vi "虚拟辐射监测仪-35-全屏版.vi"() -> ()   [LabVIEW 2013]
uses:
  <vilib>/registry/registry.llb/Registry RtKey.ctl
  <vilib>/Utility/xml.llb/Read From XML File(string).vi
  <vilib>/Instr/_visa.llb/VISA Configure Serial Port (Instr).vi
  <vilib>/Utility/inputDevices.llb/closeMouse.vi
  <vilib>/Utility/xml.llb/Write to XML File(string).vi
  <vilib>/Utility/inputDevices.llb/mouseAcquire.vi
  <vilib>/registry/registry.llb/Write Registry Value Simple STR.vi
  <vilib>/Utility/miscctls.llb/LVPoint32TypeDef.ctl
  <vilib>/Utility/miscctls.llb/LVPositionTypeDef.ctl
  <vilib>/Utility/miscctls.llb/LVBoundsTypeDef.ctl
panel:
  in  "实时数据":i32[](listbox)
  out "全探头窗口":refnum<vi>
  in  "更新列表？":bool
  out "测量值":dbl[](array[numeric])
  in  "切换窗口":bool
  in  "回复背景色标志":bool
  in  "等待时间（毫秒）":u32=10
  in  "T:G,F:B":bool
  in  "确认COM":bool
  in  "device ID":refnum<k1> caption="设备ID"
  in  "信号-弹窗选COM":bool
  out "菜单项":T1(ring)=enum."禁用"
  out "内容区域边界":T2
  out "内容区域位置":T3
  out "坐标":T4
  in  "开机启动":bool
  in  "收回":bool
  out "提示语":string
  in  "修改完成":bool=TRUE
  in  "变了？":bool
  out "编辑前项名":string[][](array[string])
  out "FREE":bool=TRUE
  in  "探头启用状态？":bool[](array[boolean])
  in  "报警记录标志？":bool[](array[boolean])
  in  "最大报警值":dbl[](array[numeric])
  in  "异常保存记录？":bool[](array[boolean])
  in  "发送次数":u8[](array[numeric])
  in  "暂停发送":bool=TRUE
  in  "探头地址":i32[](array[numeric])
  in  "备注信息":string[](array[string])
  in  "报警限值":dbl[](array[numeric])
  in  "报警状态？":bool[](array[boolean])
  out "退出":bool
  in  "波特率":enum16{"4800", "9600", "19200"}(ring)=enum."9600"
  out "报警记录":i32(listbox)
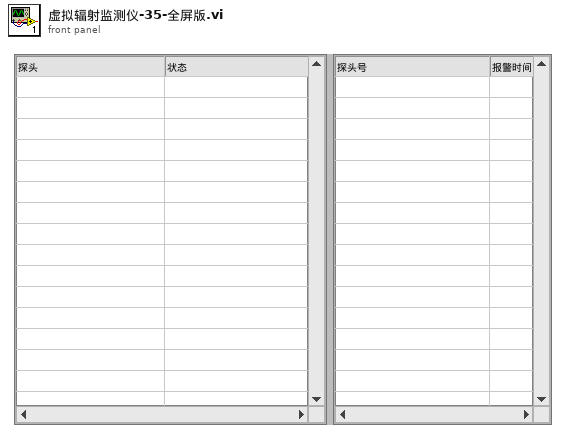
[diagram p1: front panel]
types:
  T1 = enum16{"启用", "禁用", "修改备注", "修改报警限值", "微调测量值", "探头排序", "备注信息", "报警限值"}
  T2 = typedef "LVBoundsTypeDef.ctl" = cluster{"Width":u32, "Height":u32}
  T3 = typedef "LVPositionTypeDef.ctl" = cluster{"Left":i32, "Top":i32}
  T4 = typedef "LVPoint32TypeDef.ctl" = cluster{"Horizontal":i32, "Vertical":i32}
  T5 = enum16{"初始化", "扫描探头", "发送命令", "接收数据", "暂停发送", "结束程序", "退出"}
  T6 = enum16{"启用", "禁用", "修改备注", "修改报警限值", "微调测量值", "探头排序", "备注信息"}
  T7 = enum32{"Invalid", "Standard", "Closed", "Hidden", "Minimized", "Maximized"}
  T8 = cluster{"测量值":refnum<vi>, "备注信息":refnum<vi>, "报警状态？":refnum<vi>, "探头启用状态？":refnum<vi>, "更新列表？":refnum<vi>}
  T9 = typedef "Registry RtKey.ctl" = enum32{"HKEY_CLASSES_ROOT", "HKEY_CURRENT_USER", "HKEY_LOCAL_MACHINE", "HKEY_USERS", "HKEY_PERFORMANCE_DATA", "HKEY_CURRENT_CONFIG", "HKEY_DYN_DATA"}
  T10 = cluster{"button 1":bool, "button 2":bool, "button 3":bool, "button 4":bool}
  T11 = typedef "LVRowAndColumnTypeDef.ctl" = cluster{"Row":i32, "Column":i32}
  T12 = cluster{"VISA":refnum<visa-resource-name>, "探头地址":i32[], "最大报警值":dbl[], "报警记录标志？":bool[], "报警状态？":bool[], "异常保存记录？":bool[], "报警限值":dbl[], "备注信息":string[], "探头启用状态？":bool[]}
  T13 = typedef "Registry refnum.ctl" = refnum<k1>
  T14 = cluster{"COM":refnum<visa-resource-name>, "探头地址":i32[], "探头启用状态？":bool[], "报警限值":dbl[], "开机启动？":bool, "备注信息":string[]}
  T15 = cluster{"COM":refnum<visa-resource-name>, "探头地址":i32[], "探头启用状态？":bool[], "开机启动？":bool, "探头信息":string[], "限值":cluster{"限值1":dbl, "限值2":dbl}[]}
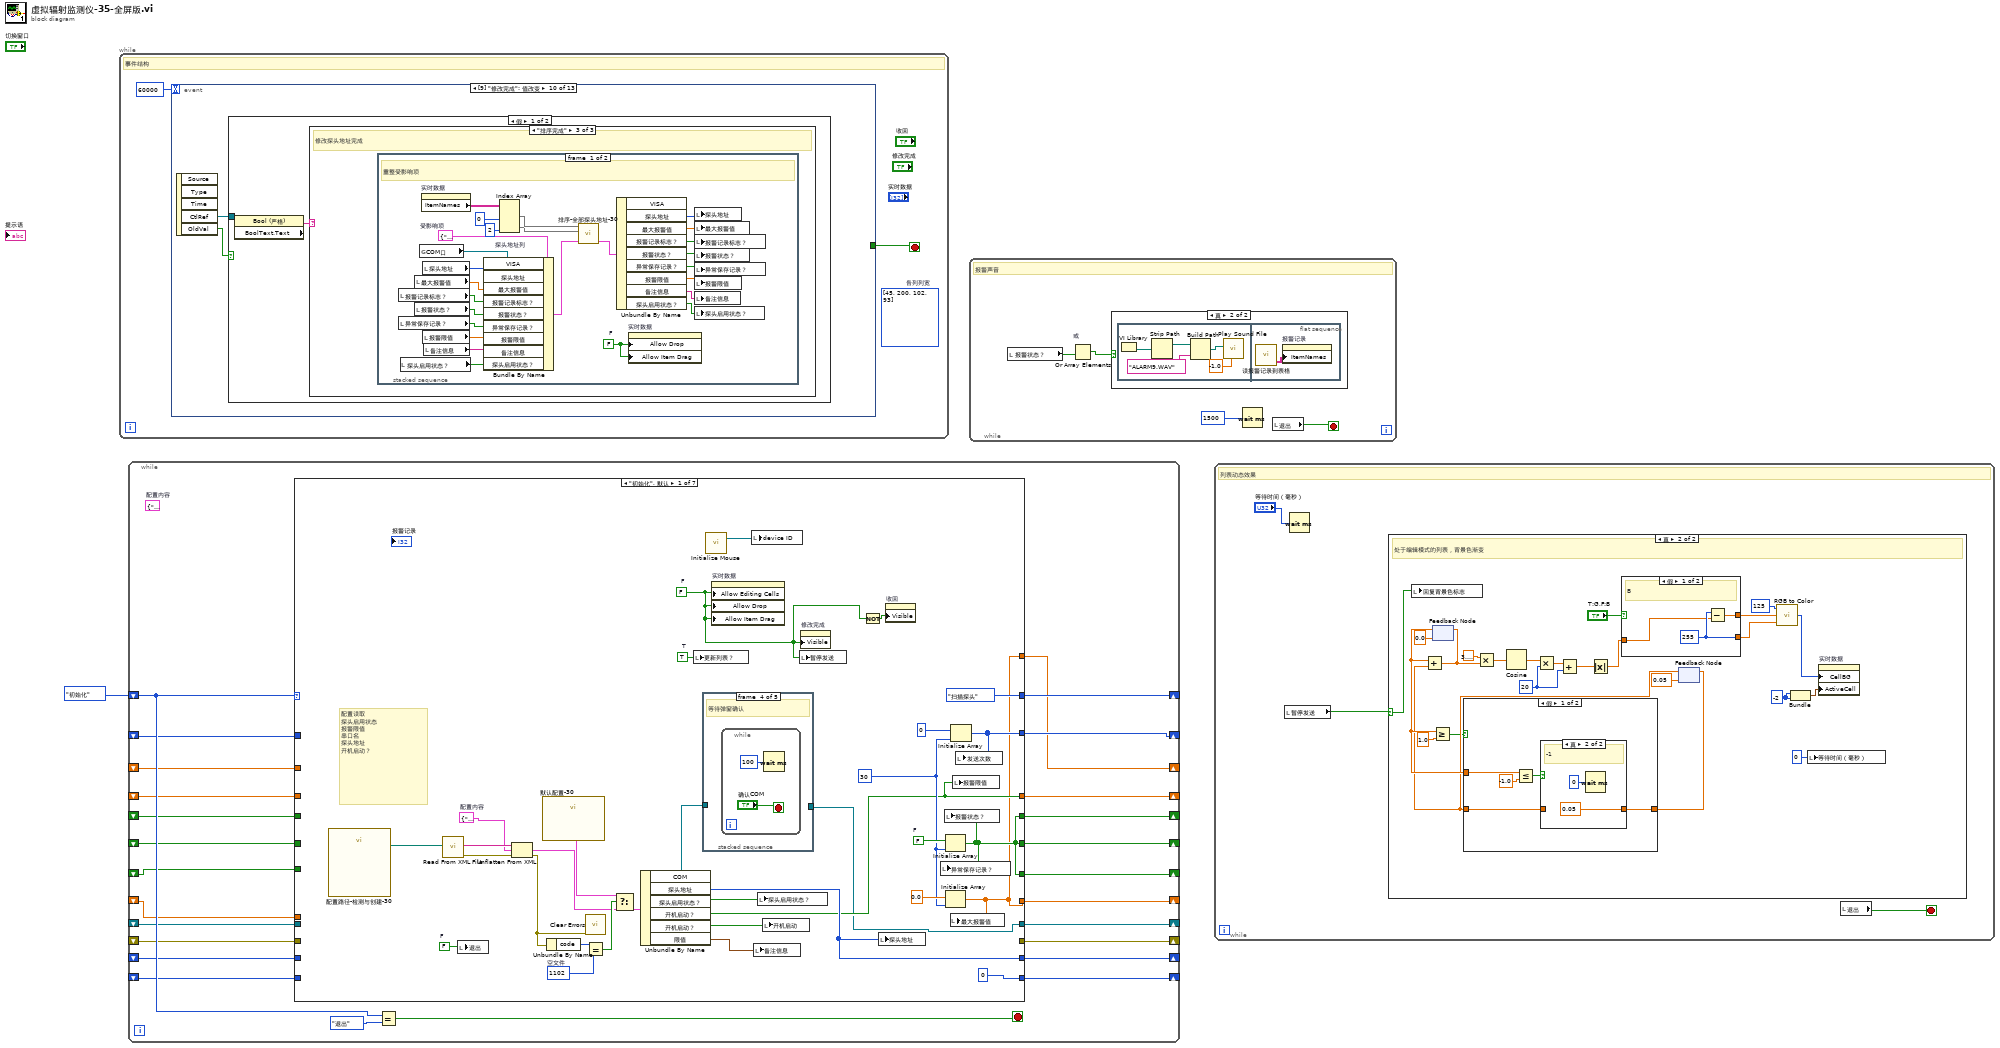
[diagram p0: block diagram]
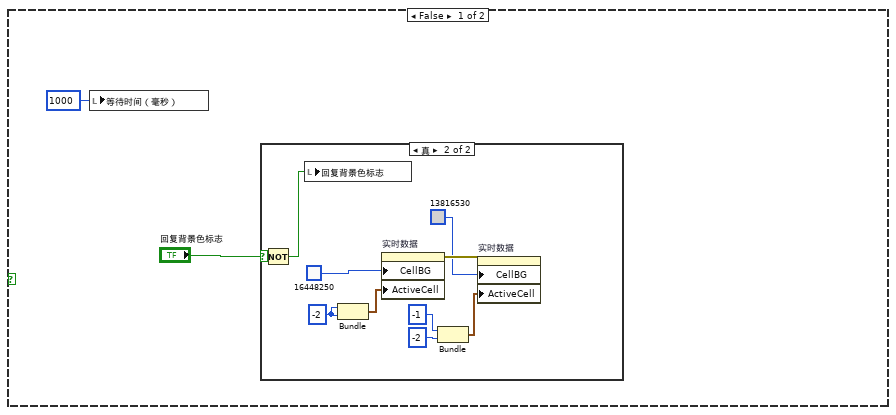
[diagram p2: hidden frame]
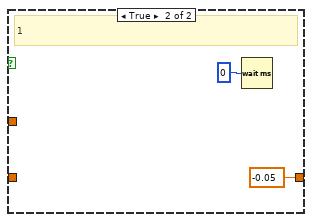
[diagram p5: hidden frame]
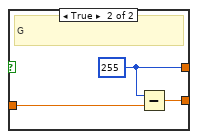
[diagram p6: hidden frame]
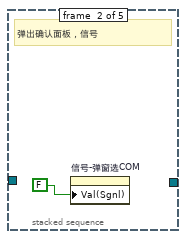
[diagram p8: hidden frame]
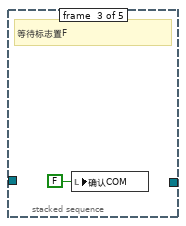
[diagram p9: hidden frame]
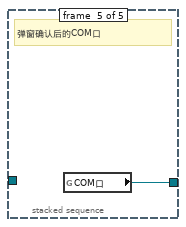
[diagram p10: hidden frame]
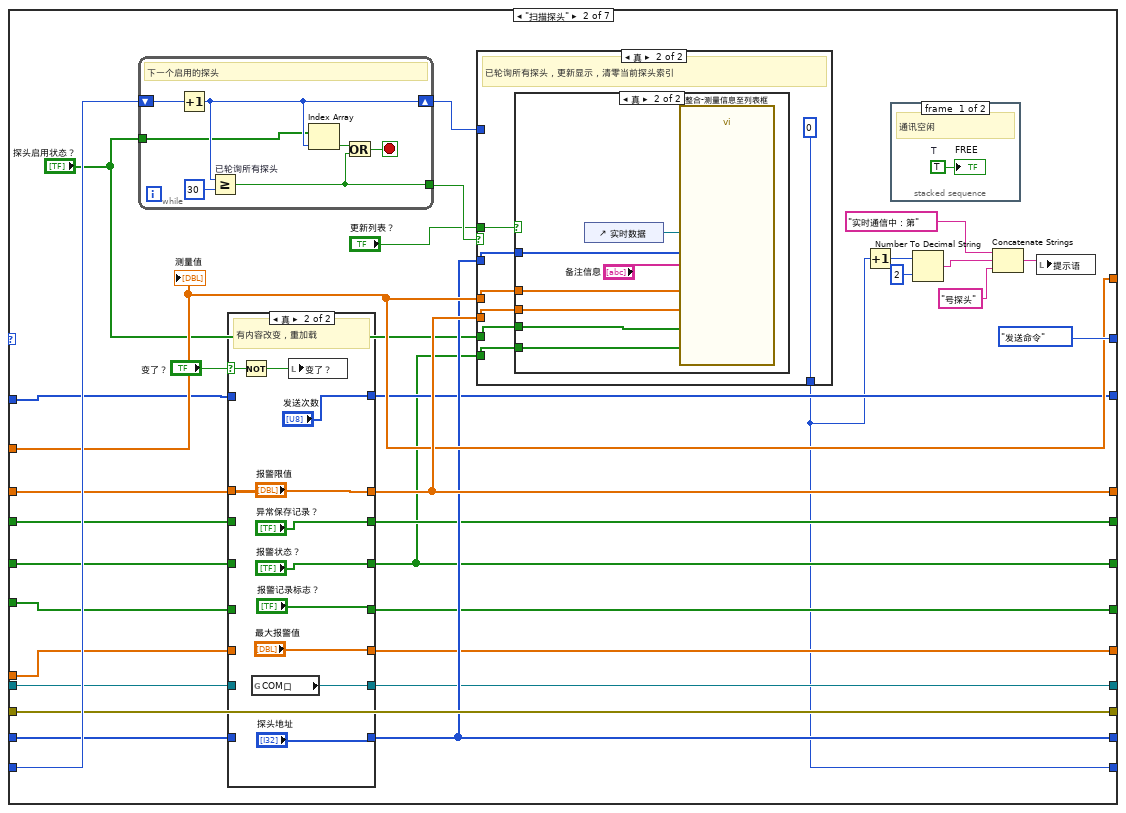
[diagram p11: hidden frame]
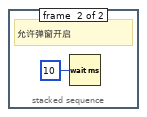
[diagram p13: hidden frame]
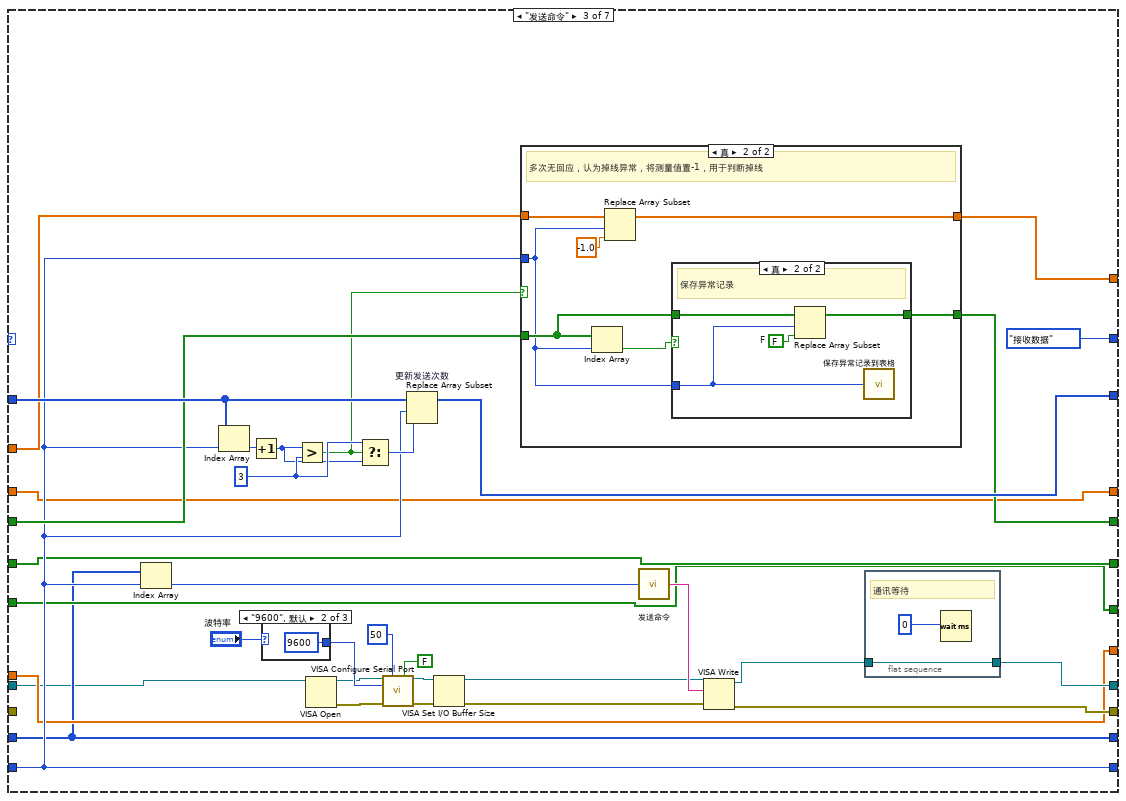
[diagram p16: hidden frame]
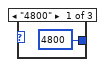
[diagram p19: hidden frame]
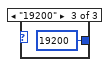
[diagram p20: hidden frame]
diagram:
  n1 = while {
    stop <- w3 stop-if-true
    (unwired) i32[] [45, 200, 102, 93]  # 各列列宽
    # "事件结构"
    n2 = event shown="[9] \"修改完成\": 值改变" {
      selector: _ -> [_ _ _ _ _ _ _ _ _ _ _ _ _]
      dyn-events: _ -> [_ _ _ _ _ _ _ _ _ _ _ _ _]
      timeout: 60000 -> [_ _ _ _ _ _ _ _ _ _ _ _ _]
      tunnel: [_ w4 _ _ _ _ _ _ _ _ _ _ _] -> w3
      event Timeout {
        n3 = event-data() -> ()  [unwired: 1 in, 2 out]
      }
      event Panel Close? {
        w4 = TRUE  # T
        n4 = event-data() -> ()  [unwired: 1 in, 4 out]
        n5 = event-data("Discard?"=w4) -> ()  [unwired: 1 in, 1 out]
        "退出" <- w4
      }
      event "信号-弹窗选COM": Value Change {
        n6 = event-data() -> ()  [unwired: 1 in, 6 out]
        n7 = flat-sequence {
          frame #0 {
            n8 = global read "全局变量-35点监测.vi" "COM口"() -> (w5:refnum<visa-resource-name>)
            n9 = control-ref of="本VI"() -> (w6:refnum<vi>)
            n10 = call "弹窗-提示选择Com口-30.vi"("VI引用句柄"=w6, "VISA资源名称"=w5) -> ()  [unwired: 9 in, 1 out]
          }
          frame #1 {
            n11 = local write "确认COM"(TRUE ("确认COM")) -> ()
          }
        }
      }
      event "实时数据": Mouse Move {
        # "注意：多列列表框一旦移动过\n就要重新定位坐标分界值"
        # "调试用"
        n12 = event-data() -> ("Coords"=w8:T4)  [unwired: 1 in, 4 out]
        n13 = disable-structure shown="禁用" {
          disable-tunnel: w8 -> [w11 _]
          frame Disabled {
            n14 = property on="实时数据" class="MCListbox (严格)"() -> ("ContentRectPos"=→"内容区域位置":T3, "ContentRectBounds"=→"内容区域边界":T2)  [unwired: 2 in, 2 out]
            "坐标" <- w11
          }
          frame Enabled {
          }
        }
      }
      event "实时数据": Mouse Down {
        # "使  右击行  列表能够获取焦点"
        n15 = event-data() -> ("Coords.Vertical"=w15:i32, "CtlRef"=w16:refnum<vi>)  [unwired: 1 in, 6 out]
        n16 = call-poly <vilib>:"Acquire Input Data.vi"("device ID"="device ID") -> ("button info"=w14:T10)  [unwired: 15 in, 3 out]
        n17 = Unbundle By Name(w14) -> ("button 2"=w13:bool)
        n18 = case shown="真" w13 {
          tunnel: w16 -> [_ w30]
          tunnel: w15 -> [_ w28]
          frame False {
          }
          frame True {
            w18 = TRUE  # T
            w26 = 20  # 行高
            # "右键"
            n19 = property class="多列列表框 (严格)"(reference=w30) -> ("ContentRectPosTop"=w29:i32)  [unwired: 1 in, 2 out]
            n20 = Subtract(x=w28, y=w29) -> (x-y=w27:i32)
            n21 = local read "实时数据"() -> (w19:i32[])
            n22 = Divide(x=w27, y=w26) -> (x/y=w25:dbl)
            n23 = Round Toward +Infinity(x=w25) -> (ceil(x): smallest int >= x=w24:dbl)
            n24 = To Long Integer(number=w24) -> (32bit integer=w22:i32)
            n25 = Subtract(x=w22, y=2 ("x")) -> (x-y=w20:i32)
            n26 = Build Array(w20) -> (w23:i32[])
            n27 = for {
              tunnel: w20 -> [w34]
              tunnel: w19 -> [w35] mode=indexing
              shift-right: [w31] -> w17
              shift-left: w18 -> [w32]
              stop <- w31 continue-if-true
              # "在选中项之外？"
              n28 = Not Equal?(x=w34, y=w35) -> (x != y?=w33:bool)
              n29 = And(x=w33, y=w32) -> (x .and. y?=w31:bool)
            }
            n30 = case shown="真" w17 {
              tunnel: w23 -> [_ w36]
              frame False {
                # "在已选中中，不赋值"
              }
              frame True {
                # "在选中项之外，赋值"
                n31 = local write "实时数据"(w36) -> ()
              }
            }
          }
        }
      }
      event "实时数据": Double Click {
        # "使 双击 可寻找到对应的列，并触发菜单处理事件，使打开修改弹窗"
        n32 = event-data() -> ("CtlRef"=w39:refnum<vi>, "Coords"=w40:T4)  [unwired: 1 in, 7 out]
        n33 = invoke class="多列列表框 (严格)" method="Point To Row Column"(reference=w39, "Point"=w40) -> ("CellPosition"=w38:T11)  [unwired: 5 in, 6 out]
        n34 = Unbundle By Name(w38) -> ("Column"=w37:i32)
        n35 = case shown="1" w37 {
          tunnel: [w42 T6."修改备注" ("菜单项") T6."微调测量值" ("菜单项") T6."修改报警限值" ("菜单项")] -> w41
          frame 0, Default {
            # "双击 探头地址列，禁用或启用"
            n36 = local read "探头启用状态？"() -> (w48:bool[])
            n37 = local read "实时数据"() -> (w47:i32[])
            n38 = Index Array(array=w47) -> (element=w46:i32)  [unwired: 1 in]
            n39 = Index Array(array=w48, index=w46) -> (element=w45:bool)
            n40 = Select(t=T6."禁用" ("菜单项"), s=w45, f=T6."启用" ("菜单项")) -> (s? t:f=w42:T6)
          }
          frame 1 {
            # "双击备注信息列，修改备注"
          }
          frame 2 {
            # "双击测量值列，微调探头"
          }
          frame 3 {
            # "双击报警限值列，修改限值"
          }
        }
        n41 = property on="菜单项" class="Enum (严格)"("Val(Sgnl)"=w41) -> ()  [unwired: 2 in, 2 out]
      }
      event "实时数据": Shortcut Menu Activation? {
        w58 = "修改备注" ("项名称")
        w61 = "禁用" ("项名称")
        w62 = "启用" ("项名称")
        n42 = event-data() -> ("CtlRef"=w70:refnum<vi>, "MenuRef"=w68:refnum<k9>)  [unwired: 1 in, 5 out]
        n43 = property class="多列列表框 (严格)"(reference=w70) -> ("Value"=w54:i32[])  [unwired: 1 in, 2 out]
        n44 = Array Size(array=w54) -> (size(s)=w56:i32)
        n45 = Equal?(x=w56, y=1) -> (x = y?=w63:bool)
        n46 = case shown="真" w63 {
          tunnel: [w72 w73] -> w65
          tunnel: [w72 w76] -> w64
          tunnel: w54 -> [_ w75]
          tunnel: [w71 w73] -> w57
          frame False {
            w72 = TRUE  # T
            # "多线选择"
            n47 = Not(x=w72) -> (.not. x?=w71:bool)
          }
          frame True {
            # "单项选择"
            n48 = local read "探头启用状态？"() -> (w77:bool[])
            n49 = Index Array(array=w75) -> (element=w74:i32)  [unwired: 1 in]
            n50 = Index Array(array=w77, index=w74) -> (element=w73:bool)
            n51 = Not(x=w73) -> (.not. x?=w76:bool)
          }
        }
        n52 = Set Menu Item Info(7:w62, 9:w64, 10:w62, 11:w68) -> (0:w67:errorcluster, 3:w66:refnum<k9>)  [unwired: 3 in]
        n53 = Set Menu Item Info(7:w61, 8:w67, 9:w65, 10:w61, 11:w66) -> (0:w60:errorcluster, 3:w59:refnum<k9>)  [unwired: 2 in]
        n54 = Set Menu Item Info(7:w58, 8:w60, 9:w57, 10:w58, 11:w59) -> ()  [unwired: 2 in, 2 out]
        n55 = local read "暂停发送"() -> (w52:bool)
        n56 = Empty Array?(array=w54) -> (empty?=w55:bool)
        n57 = Or(x=w55, y=w52) -> (x .or. y?=w53:bool)
        n58 = event-data("Discard?"=w53) -> ()  [unwired: 1 in, 1 out]
      }
      event "实时数据": Shortcut Menu Selection (User) {
        # "不在此事件中处理菜单事件"
        n59 = event-data() -> ("ItemTag"=w79:string)  [unwired: 1 in, 7 out]
        n60 = property on="菜单项" class="Enum (严格)"() -> ("Strings []"=w80:string[])  [unwired: 2 in, 2 out]
        n61 = for {
          tunnel: w80 -> [w84] mode=indexing
          tunnel: w79 -> [w83]
          tunnel: [w81] -> w78
          i -> [w81]
          stop <- w82 stop-if-true
          # "寻找匹配项"
          n62 = Equal?(x=w84, y=w83) -> (x = y?=w82:bool)
        }
        n63 = property on="菜单项" class="Enum (严格)"("Val(Sgnl)"=w78) -> ()  [unwired: 2 in, 2 out]
      }
      event "菜单项": Value Change {
        # "用于在鼠标操作 或 菜单操作 中 触发菜单事件"
        n64 = event-data() -> ("CtlRef"=w86:refnum<vi>)  [unwired: 1 in, 4 out]
        n65 = local read "暂停发送"() -> (w85:bool)
        n66 = case shown="假" w85 {
          tunnel: w86 -> [w89 _]
          frame False {
            # "暂停发送状态下，不允许产生菜单事件"
            n67 = property class="Enum (严格)"(reference=w89) -> ("RingText.Text"=w88:string)  [unwired: 1 in, 2 out]
            n68 = local read "探头地址"() -> (w91:i32[])
            n69 = local read "实时数据"() -> (w87:i32[])
            n70 = local read "备注信息"() -> (w90:string[])
            n71 = case shown="\"修改备注\"" w88 {
              tunnel: w87 -> [w94 w101 w108 w122 w136 _ _ _ _]
              tunnel: w91 -> [_ _ w107 w121 w135 _ _ _ _]
              tunnel: w90 -> [_ _ w106 _ _ _ _ _ _]
              frame "启用" {
                # "启用探头"
                n72 = local read "探头启用状态？"() -> (w93:bool[])
                n73 = for {
                  tunnel: w94 -> [w98] mode=indexing
                  shift-right: [w95] -> w92
                  shift-left: w93 -> [w96]
                  w97 = TRUE  # T
                  n74 = Replace Array Subset "更新 探头启用状态"(array=w96, new element=w97, index=w98) -> (w95:bool[])
                }
                n75 = local write "探头启用状态？"(w92) -> ()
              }
              frame "禁用" {
                # "禁用探头"
                n76 = local read "探头启用状态？"() -> (w100:bool[])
                n77 = for {
                  tunnel: w101 -> [w105] mode=indexing
                  shift-right: [w102] -> w99
                  shift-left: w100 -> [w103]
                  w104 = FALSE  # F
                  n78 = Replace Array Subset "更新 探头启用状态"(array=w103, new element=w104, index=w105) -> (w102:bool[])
                }
                n79 = local write "探头启用状态？"(w99) -> ()
              }
              frame "修改备注" {
                # "备注 只允许单项选择"
                n80 = for {
                  tunnel: w107 -> [w116]
                  tunnel: w106 -> [w110]
                  tunnel: w108 -> [w109] mode=indexing
                  n81 = Index Array(array=w116, index=w109) -> (element=w115:i32)
                  n82 = Index Array(array=w110, index=w109) -> (element=w114:string)
                  n83 = call "创建文本2"("探头地址"=w115, "当前备注信息"=w114) -> ("Result"=w113:string)  [unwired: 12 in, 1 out]
                  n84 = call "弹窗-提示修改备注-30.vi"("信息输入"=w113) -> ("新备注"=w111:string, "确定"=w112:bool)  [unwired: 16 in, 1 out]
                  n85 = case shown="真" w112 {
                    tunnel: w111 -> [_ w119]
                    tunnel: w110 -> [_ w120]
                    tunnel: w109 -> [_ w118]
                    frame False {
                      # "取消不修改"
                    }
                    frame True {
                      # "确定则修改"
                      n86 = Replace Array Subset(array=w120, new element=w119, index=w118) -> (w117:string[])
                      n87 = local write "备注信息"(w117) -> ()
                    }
                  }
                }
              }
              frame "修改报警限值" {
                # "允许批量修改"
                n88 = stacked-sequence {
                  tunnel: w122 -> [_ w130 _]
                  tunnel: w121 -> [_ w129 _]
                  frame #0 {
                    # "等到通讯空闲"
                    n89 = while {
                      stop <- w124 stop-if-true
                      # "等到通讯空闲"
                      n90 = local read "FREE"() -> (w124:bool)
                      n91 = Wait (ms)(milliseconds to wait=u32 1 ("等待时间（毫秒）")) -> ()  [unwired: 1 out]
                    }
                  }
                  frame #1 {
                    n92 = global read "全局变量-35点监测.vi" "COM口"() -> (w125:refnum<visa-resource-name>)
                    n93 = local read "报警限值"() -> (w128:dbl[])
                    n94 = control-ref of="本VI"() -> (w127:refnum<vi>)
                    n95 = call "修改-探头报警值-30.vi"("VI引用句柄"=w127, "VISA资源名称"=w125, "限值 i"=w128, "探头地址"=w129, "探头索引（列表值）"=w130) -> (1:w126)  [unwired: 5 in, 1 out]
                    n96 = local write "报警限值"(w126) -> ()
                  }
                  frame #2 {
                    # "FREE 置 F"
                    n97 = local write "FREE"(FALSE ("FREE")) -> ()
                    n98 = local write "变了？"(TRUE ("变？报警限值")) -> ()
                  }
                }
              }
              frame "微调测量值" {
                n99 = Index Array(array=w136) -> (element=w134:i32)  [unwired: 1 in]
                n100 = Index Array(array=w135, index=w134) -> (element=w133:i32)
                n101 = stacked-sequence {
                  tunnel: w133 -> [_ w140 _]
                  frame #0 {
                    # "等到 通讯空闲"
                    n102 = while {
                      stop <- w137 stop-if-true
                      # "等到通讯空闲"
                      n103 = local read "FREE"() -> (w137:bool)
                    }
                  }
                  frame #1 {
                    # "微调"
                    n104 = global read "全局变量-35点监测.vi" "COM口"() -> (w138:refnum<visa-resource-name>)
                    n105 = control-ref of="本VI"() -> (w139:refnum<vi>)
                    n106 = call "修改-微调探头测量值-30.vi"("VI引用句柄"=w139, "探头地址"=w140, "VISA资源名称"=w138) -> ()  [unwired: 8 in, 1 out]
                  }
                  frame #2 {
                    # "FREE 置 F"
                    n107 = local write "FREE"(FALSE ("FREE")) -> ()
                  }
                }
              }
              frame "探头排序" {
                # "进入可拖拽模式"
                n108 = stacked-sequence {
                  frame #0 {
                    w143 = TRUE  # T
                    # "暂停发送"
                    n109 = local write "暂停发送"(w143) -> ()
                    n110 = local write "T:G,F:B"(TRUE ("T:G,F:B")) -> ()
                  }
                  frame #1 {
                    w145 = TRUE  # T
                    # "开始拖拽"
                    n111 = property on="修改完成" class="Bool (严格)"("Visible"=w145) -> ()  [unwired: 2 in, 2 out]
                    n112 = property on="实时数据" class="多列列表框 (严格)"("Allow Drop"=w145, "Allow Item Drag"=w145) -> ()  [unwired: 2 in, 2 out]
                    n113 = property on="修改完成" class="Bool (严格)"("BoolText.Text"="排序完成" ("布尔文本.文本")) -> ()  [unwired: 2 in, 2 out]
                  }
                  frame #2 {
                    n114 = local write "提示语"("拖拽行进行探头排序" ("提示语")) -> ()
                  }
                }
              }
              frame "备注信息" {
                # "进入可编辑模式"
                n115 = stacked-sequence {
                  frame #0 {
                    w148 = TRUE  # T
                    # "暂停发送"
                    n116 = local write "暂停发送"(w148) -> ()
                    n117 = local write "T:G,F:B"(FALSE ("T:G,F:B")) -> ()
                  }
                  frame #1 {
                    w151 = TRUE  # T
                    # "开始编辑"
                    n118 = property on="实时数据" class="MCListbox (严格)"() -> ("ItemNames"=→"编辑前项名":string[][])  [unwired: 2 in, 2 out]
                    n119 = property on="实时数据" class="多列列表框 (严格)"("Allow Editing Cells"=w151) -> ()  [unwired: 2 in, 2 out]
                    n120 = property on="修改完成" class="Bool (严格)"("BoolText.Text"="编辑完成" ("布尔文本.文本")) -> ()  [unwired: 2 in, 2 out]
                    n121 = property on="修改完成" class="Bool (严格)"("Visible"=w151) -> ()  [unwired: 2 in, 2 out]
                  }
                  frame #2 {
                    n122 = local write "提示语"("点击备注信息单元格编辑" ("提示语")) -> ()
                  }
                }
              }
              frame "报警限值" {
                # "批量修改报警限值"
              }
              frame "假", Default {
              }
            }
          }
          frame True {
            # "暂停发送状态下，不允许产生菜单事件"
          }
        }
      }
      event "修改完成": Value Change {
        n123 = event-data() -> ("CtlRef"=w154:refnum<vi>, "OldVal"=w153:bool)  [unwired: 1 in, 3 out]
        n124 = case shown="假" w153 {
          tunnel: w154 -> [w156 _]
          frame False {
            n125 = property class="Bool (严格)"(reference=w156) -> ("BoolText.Text"=w155:string)  [unwired: 1 in, 2 out]
            n126 = case shown="\"排序完成\"" w155 {
              frame "假", Default {
              }
              frame "编辑完成" {
                # "修改备注信息完成"
                n127 = stacked-sequence {
                  frame #0 {
                    w158 = FALSE  # F
                    w162 = 1 ("禁用的索引 (列)")
                    # "更改受影响项"
                    n128 = property on="实时数据" class="MCListbox (严格)"() -> (error out=w161:errorcluster, "ItemNames"=w164:string[][])  [unwired: 2 in, 1 out]
                    n129 = local read "编辑前项名"() -> (w163:string[][])
                    n130 = Index Array "备注咧"(array=w164, index (col)=w162) -> (element=w159:string[])  [unwired: 1 in]
                    n131 = Replace Array Subset(array=w163, new element=w159, index (col)=w162) -> (w160:string[][])  [unwired: 1 in]
                    n132 = local write "备注信息"(w159) -> ()
                    n133 = property on="实时数据" class="MCListbox (严格)"(error in=w161, "ItemNames"=w160) -> (error out=w157:errorcluster)  [unwired: 1 in, 1 out]
                    n134 = property on="实时数据" class="MCListbox (严格)"(error in=w157, "Allow Editing Cells"=w158) -> ()  [unwired: 1 in, 2 out]
                  }
                  frame #1 {
                    # "更改标志，使在状态机中检测到更改"
                    n135 = flat-sequence {
                      frame #0 {
                        w165 = TRUE  # T
                        n136 = local write "变了？"(w165) -> ()
                      }
                      frame #1 {
                        w167 = FALSE  # F
                        w166 = FALSE  # F
                        n137 = local write "暂停发送"(w167) -> ()
                        n138 = property on="修改完成" class="Bool (严格)"("Visible"=w166) -> ()  [unwired: 2 in, 2 out]
                      }
                    }
                  }
                }
              }
              frame "排序完成" {
                # "修改探头地址完成"
                n139 = stacked-sequence {
                  frame #0 {
                    w173 = T12 {"VISA"="", "探头地址"=[], "最大报警值"=[], "报警记录标志？"=[], "报警状态？"=[], "异常保存记录？"=[], "报警限值"=[], "备注信息"=["4号楼509", "", "", "", "", "", "", "", "", "", "", "", "", "", "", "", "", "", "", "", "", "", "", "", "", "", "", "", "", ""], "探头启用状态？"=[]}  # 受影响项
                    w191 = FALSE  # F
                    # "重整受影响项"
                    n140 = local read "报警记录标志？"() -> (w187:bool[])
                    n141 = local read "异常保存记录？"() -> (w189:bool[])
                    n142 = local read "探头启用状态？"() -> (w172:bool[])
                    n143 = local read "最大报警值"() -> (w186:dbl[])
                    n144 = local read "报警状态？"() -> (w188:bool[])
                    n145 = global read "全局变量-35点监测.vi" "COM口"() -> (w169:refnum<visa-resource-name>)
                    n146 = property on="实时数据" class="MCListbox (严格)"() -> ("ItemNames"=w193:string[][])  [unwired: 2 in, 2 out]
                    n147 = local read "探头地址"() -> (w185:i32[])
                    n148 = local read "报警限值"() -> (w190:dbl[])
                    n149 = local read "备注信息"() -> (w176:string[])
                    n150 = Bundle By Name(cluster=w173, "VISA"=w169, "探头地址"=w185, "最大报警值"=w186, "报警记录标志？"=w187, "报警状态？"=w188, "异常保存记录？"=w189, "报警限值"=w190, "备注信息"=w176, "探头启用状态？"=w172) -> (w184:T12)
                    n151 = Index Array "探头地址列"(array=w193, index (col) #1=0 ("禁用的索引 (列)"), index (col) #2=2 ("索引 (列)")) -> (element #1=w175:string[], element #2=w174:string[])  [unwired: 2 in]
                    n152 = call "排序-全部探头地址-30.vi"("受影响项i"=w184, "备注信息列"=w174, "探头序号列"=w175) -> ("受影响项o"=w183:T12)  [unwired: 8 in]
                    n153 = Unbundle By Name(w183) -> ("探头地址"=w182:i32[], "最大报警值"=w181:dbl[], "报警记录标志？"=w180:bool[], "报警状态？"=w179:bool[], "异常保存记录？"=w178:bool[], "报警限值"=w177:dbl[], "备注信息"=w171:string[], "探头启用状态？"=w170:bool[])  [unwired: 1 out]
                    n154 = property on="实时数据" class="多列列表框 (严格)"("Allow Drop"=w191, "Allow Item Drag"=w191) -> ()  [unwired: 2 in, 2 out]
                    n155 = local write "备注信息"(w171) -> ()
                    n156 = local write "探头启用状态？"(w170) -> ()
                    n157 = local write "探头地址"(w182) -> ()
                    n158 = local write "最大报警值"(w181) -> ()
                    n159 = local write "报警记录标志？"(w180) -> ()
                    n160 = local write "报警状态？"(w179) -> ()
                    n161 = local write "异常保存记录？"(w178) -> ()
                    n162 = local write "报警限值"(w177) -> ()
                  }
                  frame #1 {
                    # "更改标志，使在状态机中检测到更改"
                    n163 = flat-sequence {
                      frame #0 {
                        w194 = TRUE  # T
                        n164 = local write "变了？"(w194) -> ()
                      }
                      frame #1 {
                        w196 = FALSE  # F
                        w195 = FALSE  # F
                        n165 = local write "暂停发送"(w196) -> ()
                        n166 = property on="修改完成" class="Bool (严格)"("Visible"=w195) -> ()  [unwired: 2 in, 2 out]
                      }
                    }
                  }
                }
              }
            }
          }
          frame True {
          }
        }
      }
      event "切换窗口": Value Change {
        n167 = event-data() -> ("OldVal"=w197:bool)  [unwired: 1 in, 5 out]
        n168 = case shown="真" w197 {
          frame False {
          }
          frame True {
            # "切换到大窗口浏览模式"
            n169 = control-ref of="探头启用状态？"() -> (w205:refnum<vi>)
            n170 = control-ref of="更新列表？"() -> (w198:refnum<vi>)
            n171 = control-ref of="本VI"() -> (w201:refnum<vi>)
            n172 = control-ref of="测量值"() -> (w219:refnum<vi>)
            n173 = control-ref of="备注信息"() -> (w218:refnum<vi>)
            n174 = control-ref of="报警状态？"() -> (w217:refnum<vi>)
            n175 = Bundle By Name(cluster=T8 {"测量值"=refnum, "备注信息"=refnum, "报警状态？"=refnum, "探头启用状态？"=refnum, "更新列表？"=refnum}, "测量值"=w219, "备注信息"=w218, "报警状态？"=w217, "更新列表？"=w198, "探头启用状态？"=w205) -> (w215:T8)
            n176 = vi-ref "探头模块-精简版.vi"() -> (w216:refnum<vi>)
            n177 = invoke on="传入引用" class="VI" method="Ctrl Val.Set"(reference=w216, "Control Name"="引用传入" ("控件名"), "Value"=w215) -> (reference out=w211:refnum<vi>, error out=w209:errorcluster)  [unwired: 2 in, 3 out]
            n178 = local write "更新列表？"(FALSE ("更新列表？")) -> ()
            n179 = invoke on="运行VI" class="VI" method="Run VI"(reference=w211, error in=w209, "Wait until done"=FALSE ("结束前等待"), "Auto Dispose Ref"=TRUE ("自动销毁引用")) -> (reference out=w210:refnum<vi>, error out=w206:errorcluster)  [unwired: 1 in, 3 out]
            n180 = invoke on="打开前面板" class="VI" method="FP.Open"(reference=w210, error in=w206, "Activate"=TRUE ("激活？"), "State"=T7."Standard" ("状态")) -> (reference out=→"全探头窗口":refnum<vi>, error out=w204:errorcluster)  [unwired: 1 in, 3 out]
            n181 = property class="VI"(reference=w201, error in=w204, "FP.State"=T7."Hidden" ("前面板窗口:状态")) -> (error out=w203:errorcluster)  [unwired: 1 out]
            n182 = call <vilib>:"Clear Errors.vi"("error in (no error)"=w203) -> ()  [unwired: 6 in, 1 out]
          }
        }
      }
      event "更新列表？": Value Change {
        n183 = event-data() -> ()  [unwired: 1 in, 6 out]
        n184 = local read "全探头窗口"() -> (w227:refnum<vi>)
        n185 = control-ref of="本VI"() -> (w224:refnum<vi>)
        n186 = disable-structure shown="启用" {
          disable-tunnel: w227 -> [w230 w231]
          disable-tunnel: [w229 w231] -> w226
          disable-tunnel: [w228 _] -> w225
          frame Disabled {
            n187 = invoke class="VI" method="Abort VI"(reference=w230) -> (reference out=w229:refnum<vi>, error out=w228:errorcluster)  [unwired: 2 in, 1 out]
          }
          frame Enabled {
          }
        }
        n188 = invoke class="VI" method="FP.Close"(reference=w226, error in=w225) -> (error out=w222:errorcluster)  [unwired: 1 in, 2 out]
        n189 = property class="VI"(reference=w224, error in=w222, "FP.State"=T7."Standard" ("前面板窗口:状态")) -> (error out=w221:errorcluster)  [unwired: 1 out]
        n190 = call <vilib>:"Clear Errors.vi"("error in (no error)"=w221) -> ()  [unwired: 6 in, 1 out]
      }
      event "开机启动": Value Change {
        n191 = event-data() -> ()  [unwired: 1 in, 5 out]
        n192 = case shown="真" "开机启动" {
          frame False {
            n193 = call <vilib>:"Open Registry Key.vi"("subkey"="SOFTWARE\\Microsoft\\Windows\\CurrentVersion\\Run", "root key (HKEY_LOCAL_MACHINE)"=Registry_RtKey."HKEY_LOCAL_MACHINE") -> ("error out"=w238:errorcluster, "refnum out"=w239:T13)  [unwired: 8 in]
            n194 = call <vilib>:"Delete Registry Value.vi"("error in (no error)"=w238, "value"="6103J-16", "refnum"=w239) -> ("error out"=w237:errorcluster, "refnum out"=w236:T13)  [unwired: 7 in]
            n195 = call <vilib>:"Close Registry Key.vi"("error in (no error)"=w237, "refnum"=w236) -> ("error out"=w233:errorcluster)  [unwired: 5 in]
            n196 = call <vilib>:"Simple Error Handler.vi"("error in (no error)"=w233) -> ()  [unwired: 4 in, 5 out]
          }
          frame True {
            n197 = VI Library() -> (path=w243:path)
            n198 = Strip Path(path=w243) -> (stripped path=w245:path)  [unwired: 1 out]
            n199 = call <vilib>:"Create Registry Key.vi"("subkey"="SOFTWARE\\Microsoft\\Windows\\CurrentVersion\\Run", "root key (HKEY_LOCAL_MACHINE)"=Registry_RtKey."HKEY_LOCAL_MACHINE") -> ("refnum out"=w252:T13)  [unwired: 7 in, 2 out]
            n200 = Build Path(base path=w245, name or relative path="核辐射在线测量16路.exe" ("读报警文件")) -> (appended path=w242:path)
            n201 = Path To String(path=w242) -> (string=w241:string)
            n202 = call-poly <vilib>:"Write Registry Value Simple.vi"("String/Binary data"=w241, "simple data type"=enum16{"String", "Binary", "DWORD"}."String", "value"="6103J-16", "refnum"=w252) -> ("error out"=w247:errorcluster, "refnum out"=w248:T13)  [unwired: 4 in]
            n203 = call <vilib>:"Close Registry Key.vi"("error in (no error)"=w247, "refnum"=w248) -> ("error out"=w249:errorcluster)  [unwired: 5 in]
            n204 = call <vilib>:"Simple Error Handler.vi"("error in (no error)"=w249) -> ()  [unwired: 4 in, 5 out]
          }
        }
      }
    }
  }
  n205 = while {
    shift-right: [w277] -> _
    shift-left: T5."初始化" -> [w278]
    shift-right: [w276] -> _
    shift-left: _ -> [w274]
    shift-right: [w275] -> _
    shift-left: _ -> [w273]
    shift-right: [w258] -> _
    shift-left: _ -> [w263]
    shift-right: [w257] -> _
    shift-left: _ -> [w265]
    shift-right: [w262] -> _
    shift-left: _ -> [w264]
    shift-right: [w270] -> _
    shift-left: _ -> [w271]
    shift-right: [w254] -> _
    shift-left: _ -> [w268]
    shift-right: [w266] -> _
    shift-left: _ -> [w267]
    shift-right: [w256] -> _
    shift-left: _ -> [w261]
    shift-right: [w255] -> _
    shift-left: _ -> [w260]
    shift-right: [w259] -> _
    shift-left: _ -> [w269]
    stop <- w279 stop-if-true
    (unwired) T14 {"COM"="", "探头地址"=[], "探头启用状态？"=[], "报警限值"=[], "开机启动？"=FALSE, "备注信息"=[]}  # 配置内容
    n206 = case shown="\"初始化\", 默认" w278 {
      selector: w278 -> [_ _ _ _ _ _ w584]
      tunnel: [T5."扫描探头" T5."发送命令" T5."接收数据" T5."暂停发送" w551 T5."退出" w584] -> w277
      tunnel: [w281 w326 w401 w461 w549 _ w583] -> w276
      tunnel: [_ w347 w413 w460 w548 _ w582] -> w275
      tunnel: w274 -> [_ w327 w391 w463 w549 w569 w583]
      tunnel: w273 -> [_ w347 _ w462 w548 w571 w582]
      tunnel: w271 -> [_ w332 w408 w457 w541 w562 w578]
      tunnel: [w288 w331 w406 w451 w541 w562 w578] -> w270
      tunnel: w269 -> [_ w340 w392 w445 w535 w556 w574]
      tunnel: w268 -> [_ w348 w400 w444 w534 w555 w573]
      tunnel: w267 -> [_ w334 w405 w456 w539 w560 w575]
      tunnel: [w287 w333 w404 w450 w539 w560 w575] -> w266
      tunnel: [0 ("维数大小") w319 w400 w444 w534 w555 w573] -> w254
      tunnel: w265 -> [_ w330 w395 w458 w538 w559 w581]
      tunnel: w264 -> [_ w341 w398 w455 w542 w563 w577]
      tunnel: w263 -> [_ w342 w396 w449 w540 w561 w576]
      tunnel: [w286 w341 w397 w452 w542 w563 w577] -> w262
      tunnel: w261 -> [_ w336 w394 w454 w537 w558 w580]
      tunnel: w260 -> [_ w338 w393 w453 w536 w557 w579]
      tunnel: [w292 w339 w392 w445 w535 w556 w574] -> w259
      tunnel: [w289 w343 w396 w449 w540 w561 w576] -> w258
      tunnel: [w287 w329 w395 w447 w538 w559 w581] -> w257
      tunnel: [w287 w335 w394 w448 w537 w558 w580] -> w256
      tunnel: [w286 w337 w393 w446 w536 w557 w579] -> w255
      frame "初始化", Default {
        w280 = TRUE  # T
        w284 = FALSE  # F
        w291 = T14 {"COM"="", "探头地址"=[], "探头启用状态？"=[], "报警限值"=[], "开机启动？"=FALSE, "备注信息"=[]}  # 配置内容
        w298 = 1102  # 空文件
        w300 = 30 ("维数大小")
        w304 = FALSE  # F
        w310 = FALSE  # F
        # "配置读取\n探头启用状态\n报警限值\n串口名\n探头地址\n开机启动？"
        n207 = call "配置路径-检测与创建-30.vi"() -> ("配置文件路径"=w309:path)  [unwired: 11 in]
        n208 = call-poly <vilib>:"Read From XML File.vi"("XML File Path"=w309) -> ("error out"=w307:errorcluster, "XML Elements"=w308:string)  [unwired: 8 in, 1 out]
        n209 = local write "退出"(w310) -> ()
        n210 = Unflatten From XML(xml string=w308, type=w291, error in (no error)=w307) -> (value=w294:T14, error out=w293:errorcluster)
        n211 = call "默认配置-30.vi"() -> ("默认配置"=w295:T15)  [unwired: 11 in]
        n212 = Unbundle By Name(w293) -> ("code"=w299:i32)
        n213 = call <vilib>:"Clear Errors.vi"("error in (no error)"=w293) -> ()  [unwired: 6 in, 1 out]
        n214 = Equal?(x=w299, y=w298) -> (x = y?=w296:bool)
        n215 = Select(t=w295, s=w296, f=w294) -> (s? t:f=w297:T15)
        n216 = Unbundle By Name(w297) -> ("COM"=w282:refnum<visa-resource-name>, "探头地址"=w292:i32[], "探头启用状态？"=w305:bool[], "开机启动？"=w289:bool, "开机启动？"=w306:bool, "限值"=w290:cluster{"限值1":dbl, "限值2":dbl}[])
        n217 = local write "更新列表？"(w280) -> ()
        n218 = stacked-sequence {
          tunnel: w282 -> [_ _ _ _ _]
          tunnel: [_ _ _ _ w316] -> w281
          frame #0 {
            # "读取配置保存的COM口"
          }
          frame #1 {
            # "弹出确认面板，信号"
            n219 = property on="信号-弹窗选COM" class="Bool (严格)"("Val(Sgnl)"=FALSE ("允许编辑单元格")) -> ()  [unwired: 2 in, 2 out]
          }
          frame #2 {
            # "等待标志置F"
            n220 = local write "确认COM"(FALSE ("确认COM")) -> ()
          }
          frame #3 {
            # "等待弹窗确认"
            n221 = while {
              stop <- "确认COM" stop-if-true
              n222 = Wait (ms)(milliseconds to wait=u32 100 ("等待时间（毫秒）")) -> ()  [unwired: 1 out]
            }
          }
          frame #4 {
            # "弹窗确认后的COM口"
            n223 = global read "全局变量-35点监测.vi" "COM口"() -> (w316:refnum<visa-resource-name>)
          }
        }
        n224 = call <vilib>:"Initialize Mouse.vi"() -> ("device ID"=w285:refnum<k1>)  [unwired: 10 in, 1 out]
        n225 = property on="实时数据" class="多列列表框 (严格)"("Allow Editing Cells"=w284, "Allow Drop"=w284, "Allow Item Drag"=w284) -> ()  [unwired: 2 in, 2 out]
        n226 = local write "device ID"(w285) -> ()
        n227 = local write "备注信息"(w290) -> ()
        n228 = local write "探头启用状态？"(w305) -> ()
        n229 = local write "开机启动"(w306) -> ()
        n230 = local write "暂停发送"(w284) -> ()
        n231 = property on="修改完成" class="Bool (严格)"("Visible"=w284) -> ()  [unwired: 2 in, 2 out]
        n232 = Not(x=w284) -> (.not. x?=w283:bool)
        n233 = local write "探头地址"(w292) -> ()
        n234 = property on="收回" class="Bool (严格)"("Visible"=w283) -> ()  [unwired: 2 in, 2 out]
        n235 = Initialize Array(w304, w300) -> (w287:bool[])
        n236 = local write "异常保存记录？"(w287) -> ()
        n237 = local write "报警状态？"(w287) -> ()
        n238 = Initialize Array(0.0 ("维数大小"), w300) -> (w286:dbl[])
        n239 = local write "最大报警值"(w286) -> ()
        n240 = Initialize Array(u8 0 ("维数大小"), w300) -> (w288:u8[])
        n241 = local write "报警限值"(w289) -> ()
        n242 = local write "发送次数"(w288) -> ()
      }
      frame "扫描探头" {
        n243 = while {
          shift-right: [w386] -> w346
          shift-left: w348 -> [w390]
          tunnel: [w385] -> w318
          tunnel: "探头启用状态？" -> [w384]
          stop <- w387 stop-if-true
          # "下一个启用的探头"
          n244 = Increment(x=w390) -> (x+1=w386:i32)
          n245 = Greater Or Equal? "已轮询所有探头"(x=w386, y=u8 30) -> (x >= y?=w385:bool)
          n246 = Index Array(array=w384, index=w386) -> (element=w389:bool)
          n247 = Or(x=w389, y=w385) -> (x .or. y?=w387:bool)
        }
        n248 = case shown="真" "变了？" {
          selector: "变了？" -> [_ w365]
          tunnel: [w356 "报警限值"] -> w343
          tunnel: w342 -> [w356 _]
          tunnel: w340 -> [w355 _]
          tunnel: [w355 "探头地址"] -> w339
          tunnel: w338 -> [w354 _]
          tunnel: [w354 "最大报警值"] -> w337
          tunnel: w336 -> [w353 _]
          tunnel: [w353 "报警记录标志？"] -> w335
          tunnel: w330 -> [w352 _]
          tunnel: [w352 "报警状态？"] -> w329
          tunnel: w334 -> [w351 _]
          tunnel: [w351 "异常保存记录？"] -> w333
          tunnel: w332 -> [w350 _]
          tunnel: [w350 "发送次数"] -> w331
          tunnel: w327 -> [w349 _]
          tunnel: [w349 w357] -> w326
          frame False {
            # "没有内容改变，则传递"
          }
          frame True {
            # "有内容改变，重加载"
            n249 = Not(x=w365) -> (.not. x?=w364:bool)
            n250 = global read "全局变量-35点监测.vi" "COM口"() -> (w357:refnum<visa-resource-name>)
            n251 = local write "变了？"(w364) -> ()
          }
        }
        n252 = case shown="真" w318 {
          tunnel: w341 -> [_ w376]
          tunnel: w343 -> [_ w375]
          tunnel: w329 -> [_ w374]
          tunnel: w339 -> [_ w373]
          tunnel: w346 -> [w369 _]
          tunnel: [w369 u8 0] -> w319
          tunnel: "探头启用状态？" -> [_ w371]
          tunnel: "更新列表？" -> [_ w370]
          frame False {
            # "更新当前探头索引，通知全探头窗口更新显示"
          }
          frame True {
            # "已轮询所有探头，更新显示，清零当前探头索引"
            n253 = case shown="真" w370 {
              tunnel: w376 -> [_ w381]
              tunnel: w375 -> [_ w380]
              tunnel: w374 -> [_ w379]
              tunnel: w373 -> [_ w378]
              tunnel: w371 -> [_ w377]
              frame False {
              }
              frame True {
                n254 = control-ref of="实时数据"() -> (w383:refnum<vi>)
                n255 = call "整合-测量信息至列表框.vi"("限值"=w379, "测量值"=w377, "MCListbox引用句柄"=w383, "备注信息"=w380, "报警状态"=w381, "探头地址"="备注信息", "探头启用状态？"=w378) -> ()  [unwired: 5 in]
              }
            }
          }
        }
        n256 = Increment(x=w319) -> (x+1=w320:i32)
        n257 = stacked-sequence {
          frame #0 {
            w367 = TRUE  # T
            # "通讯空闲"
            "FREE" <- w367
          }
          frame #1 {
            # "允许弹窗开启"
            n258 = Wait (ms)(milliseconds to wait=u32 10 ("等待时间（毫秒）")) -> ()  [unwired: 1 out]
          }
        }
        n259 = Number To Decimal String(number=w320, width (-)=i16 2 ("宽度(-)")) -> (decimal integer string=w323:string)
        n260 = Concatenate Strings("实时通信中：第" ("字符串"), w323, "号探头" ("字符串")) -> (w325:string)
        n261 = local write "提示语"(w325) -> ()
        "测量值" <- w341
      }
      frame "发送命令" {
        w411 = 3
        n262 = Index Array(array=w392, index=w400) -> (element=w399:i32)
        n263 = Index Array(array=w408, index=w400) -> (element=w410:u8)
        n264 = Increment(x=w410) -> (x+1=w409:u8)
        n265 = case shown="\"9600\", 默认" "波特率" {
          tunnel: [u16 4800 u16 9600 u16 19200] -> w423
          frame "4800" {
          }
          frame "9600", Default {
          }
          frame "19200" {
          }
        }
        n266 = Greater?(x=w409, y=w411) -> (0:w403:bool)
        n267 = VISA Open(VISA resource name=w391) -> (VISA resource name=w414:refnum<visa-resource-name>, error out=w415:errorcluster)  [unwired: 1 in, 3 out]
        n268 = Select(t=w411, s=w403, f=w409) -> (s? t:f=w407:i32)
        n269 = call-poly "VISA Configure Serial Port"("VISA resource name"=w414, "timeout (10sec)"=u32 50, "Enable Termination\nChar (T)"=FALSE ("Enable Termination\nChar (T)"), "baud rate (9600)"=w423, "error in (no error)"=w415) -> ("VISA resource name out"=w416:refnum<visa-resource-name>, "error out"=w417:errorcluster)  [unwired: 3 in, 6 out]
        n270 = Replace Array Subset "更新发送次数"(array=w408, new element=w407, index=w400) -> (w406:u8[])
        n271 = VISA Set I/O Buffer Size(VISA resource name=w416, error in (no error)=w417) -> (VISA resource name out=w418:refnum<visa-resource-name>, error out=w419:errorcluster)  [unwired: 2 out]
        n272 = case shown="真" w403 {
          tunnel: w405 -> [w428 w434]
          tunnel: [w428 w433] -> w404
          tunnel: w400 -> [_ w431]
          tunnel: w398 -> [w427 w432]
          tunnel: [w427 w429] -> w397
          frame False {
            # "通信正常"
          }
          frame True {
            # "多次无回应，认为掉线异常，将测量值置-1，用于判断掉线"
            n273 = Index Array(array=w434, index=w431) -> (element=w435:bool)
            n274 = Replace Array Subset(array=w432, new element=-1.0 ("新元素/子数组"), index=w431) -> (w429:dbl[])
            n275 = case shown="真" w435 {
              tunnel: w431 -> [_ w439]
              tunnel: w434 -> [w436 w440]
              tunnel: [w436 w437] -> w433
              frame False {
              }
              frame True {
                w438 = FALSE  # F
                # "保存异常记录"
                n276 = Replace Array Subset(array=w440, new element=w438, index=w439) -> (w437:bool[])
                n277 = call "保存异常记录到表格.vi"("探头号"=w439) -> ()  [unwired: 1 in]
              }
            }
          }
        }
        n278 = call "发送命令.vi"("探头号"=w399) -> ("探头命令"=w424:string)
        n279 = VISA Write(VISA resource name=w418, write buffer=w424, error in (no error)=w419) -> (VISA resource name out=w402:refnum<visa-resource-name>, error out=w413:errorcluster)  [unwired: 1 out]
        n280 = flat-sequence {
          tunnel: w402 -> [w426]
          tunnel: [w426] -> w401
          frame #0 {
            # "通讯等待"
            n281 = Wait (ms)(milliseconds to wait=u32 0 ("毫秒倍数")) -> ()  [unwired: 1 out]
          }
        }
      }
      frame "接收数据" {
        n282 = VISA Read(VISA resource name=w463, byte count=u32 9 ("字节总数"), error in (no error)=w462) -> (VISA resource name out=w461:refnum<visa-resource-name>, read buffer=w464:string, error out=w460:errorcluster)  [unwired: 1 out]
        n283 = String To Byte Array(string=w464) -> (unsigned byte array=w466:u8[])
        n284 = call "数据验证处理.vi"("接收数组"=w466) -> ("测量值"=w468:dbl, "布尔"=w467:bool)  [unwired: 1 out]
        n285 = case shown="真" w467 {
          tunnel: w468 -> [_ w475]
          tunnel: w444 -> [_ w488]
          tunnel: w458 -> [w471 w493]
          tunnel: w457 -> [w473 w492]
          tunnel: w456 -> [w472 w491]
          tunnel: w455 -> [w474 w490]
          tunnel: w449 -> [_ w489]
          tunnel: w454 -> [w470 w487]
          tunnel: w453 -> [w469 w486]
          tunnel: w445 -> [_ w485]
          tunnel: [w474 w481] -> w452
          tunnel: [w473 w480] -> w451
          tunnel: [w472 w479] -> w450
          tunnel: [w470 w478] -> w448
          tunnel: [w471 w477] -> w447
          tunnel: [w469 w476] -> w446
          frame False {
            # "校验错误"
          }
          frame True {
            w494 = TRUE  # T
            # "CRC 校验正确"
            n286 = Index Array "读 限值"(array=w489, index=w488) -> (element=w483:dbl)
            n287 = Replace Array Subset "更新 异常保存？"(array=w491, new element=w494, index=w488) -> (w479:bool[])
            n288 = Replace Array Subset "更新 发送次数"(array=w492, new element=0, index=w488) -> (w480:u8[])
            n289 = Replace Array Subset "更新 测量值"(array=w490, new element=w475, index=w488) -> (w481:dbl[])
            n290 = Index Array "读 报警记录标志"(array=w487, index=w488) -> (element=w482:bool)
            n291 = Greater Or Equal?(x=w475, y=w483) -> (x >= y?=w484:bool)
            n292 = Replace Array Subset "更新 报警状态"(array=w493, new element=w484, index=w488) -> (w477:bool[])
            n293 = case shown="真" w484 {
              tunnel: w475 -> [_ w508]
              tunnel: w482 -> [_ w507]
              tunnel: w486 -> [w496 w506]
              tunnel: w488 -> [w498 w505]
              tunnel: w485 -> [_ w504]
              tunnel: w487 -> [w499 w503]
              tunnel: [w497 w502] -> w478
              tunnel: [w496 w501] -> w476
              frame False {
                w500 = FALSE  # F
                # "未发生报警"
                n294 = Replace Array Subset "更新 报警记录标志"(array=w499, new element=w500, index=w498) -> (w497:bool[])
              }
              frame True {
                # "发生报警"
                n295 = case shown="真" w507 {
                  tunnel: w508 -> [w516 w524]
                  tunnel: w506 -> [w517 w521]
                  tunnel: w505 -> [w512 w522]
                  tunnel: w504 -> [w514 w520]
                  tunnel: w503 -> [w513 w518]
                  tunnel: [w510 w518] -> w502
                  tunnel: [w509 w519] -> w501
                  frame False {
                    w511 = TRUE  # T
                    # "刚进入报警状态，开始更新最大报警值 并记录"
                    n296 = Index Array "读 探头地址"(array=w514, index=w512) -> (element=w515:i32)
                    n297 = Replace Array Subset "更新 最大报警值"(array=w517, new element=w516, index=w512) -> (w509:dbl[])
                    n298 = call "保存报警记录到表格.vi"("报警值"=w516, "探头号"=w515) -> ()  [unwired: 1 in]
                    n299 = Replace Array Subset "更新 报警记录标志"(array=w513, new element=w511, index=w512) -> (w510:bool[])
                  }
                  frame True {
                    # "已在报警状态中，判断新测量值与最大报警值关系"
                    n300 = Index Array "读 最大报警值"(array=w521, index=w522) -> (element=w523:dbl)
                    n301 = Greater?(x=w524, y=w523) -> (0:w525:bool)
                    n302 = case shown="真" w525 {
                      tunnel: w524 -> [_ w531]
                      tunnel: w522 -> [_ w529]
                      tunnel: w521 -> [w526 w532]
                      tunnel: w520 -> [_ w530]
                      tunnel: [w526 w527] -> w519
                      frame False {
                        # "没有更大的报警值"
                      }
                      frame True {
                        # "新的最大报警值，记录"
                        n303 = Replace Array Subset "更新 最大报警值"(array=w532, new element=w531, index=w529) -> (w527:dbl[])
                        n304 = Index Array "读 探头地址"(array=w530, index=w529) -> (element=w528:i32)
                        n305 = call "保存报警记录到表格.vi"("报警值"=w531, "探头号"=w528) -> ()  [unwired: 1 in]
                      }
                    }
                  }
                }
              }
            }
          }
        }
      }
      frame "暂停发送" {
        n306 = Wait (ms)(milliseconds to wait=u32 10 ("毫秒倍数")) -> ()  [unwired: 1 out]
        n307 = local read "退出"() -> (w547:bool)
        n308 = Select(t=T5."暂停发送", s="暂停发送", f=T5."扫描探头") -> (s? t:f=w550:T5)
        n309 = Select(t=T5."结束程序", s=w547, f=w550) -> (s? t:f=w551:T5)
      }
      frame "结束程序" {
        w554 = T14 {"COM"="", "探头地址"=[], "探头启用状态？"=[], "报警限值"=[], "开机启动？"=FALSE, "备注信息"=[]}  # 配置内容
        # "配置保存\n探头启用状态\n报警限值\n串口名\n探头地址\n开机启动？"
        n310 = VISA Close(VISA resource name=w569, error in (no error)=w571) -> (error out=w572:errorcluster)
        n311 = call <vilib>:"Clear Errors.vi"("error in (no error)"=w572) -> ()  [unwired: 6 in, 1 out]
        n312 = local read "探头启用状态？"() -> (w567:bool[])
        n313 = local read "备注信息"() -> (w553:string[])
        n314 = local read "开机启动"() -> (w568:bool)
        n315 = Bundle By Name(cluster=w554, "备注信息"=w553, "COM"=w569, "探头地址"=w556, "探头启用状态？"=w567, "报警限值"=w561, "开机启动？"=w568) -> (w566:T14)
        n316 = Flatten To XML(anything=w566) -> (xml string=w565:string)
        n317 = call "配置路径-检测与创建-30.vi"() -> ("配置文件路径"=w564:path)  [unwired: 11 in]
        n318 = call-poly <vilib>:"Write to XML File.vi"("XML Input"=w565, "XML File Path"=w564) -> ()  [unwired: 7 in, 3 out]
        n319 = local read "device ID"() -> (w552:refnum<k1>)
        n320 = call-poly <vilib>:"Close Input Device.vi"("device ID"=w552) -> ()  [unwired: 9 in, 1 out]
      }
      frame "退出" {
        n321 = Quit LabVIEW() -> ()  [unwired: 1 in]
      }
    }
    n322 = Equal?(x=w278, y=T5."退出") -> (x = y?=w279:bool)
  }
  n323 = while {
    stop <- w587 stop-if-true
    # "报警声音"
    n324 = local read "报警状态？"() -> (w585:bool[])
    n325 = Or Array Elements "或"(Boolean array=w585) -> (logical OR=w586:bool)
    n326 = case shown="真" w586 {
      frame False {
      }
      frame True {
        n327 = flat-sequence {
          frame #0 {
            n328 = VI Library() -> (path=w593:path)
            n329 = Strip Path(path=w593) -> (stripped path=w592:path)  [unwired: 1 out]
            n330 = Build Path(base path=w592, name or relative path="ALARM9.WAV" ("名称或相对路径")) -> (appended path=w591:path)
            n331 = call <vilib>:"Play Sound File.vi"("timeout (sec)"=-1.0, "path"=w591) -> ()  [unwired: 8 in, 2 out]
          }
          frame #1 {
            n332 = call "读报警记录到表格.vi"() -> ("表格"=w594:string[][])  [unwired: 2 in, 1 out]
            n333 = property on="报警记录" class="MCListbox (严格)"("ItemNames"=w594) -> ()  [unwired: 2 in, 2 out]
          }
        }
      }
    }
    n334 = Wait (ms)(milliseconds to wait=u32 1500 ("毫秒倍数")) -> ()  [unwired: 1 out]
    n335 = local read "退出"() -> (w587:bool)
  }
  n336 = while {
    stop <- w596 stop-if-true
    # "列表动态效果"
    n337 = local read "暂停发送"() -> (w595:bool)
    n338 = Wait (ms)(milliseconds to wait="等待时间（毫秒）") -> ()  [unwired: 1 out]
    n339 = case shown="真" w595 {
      selector: w595 -> [_ w613]
      frame False {
        n340 = local write "等待时间（毫秒）"(u32 1000 ("等待时间（毫秒）")) -> ()
        n341 = case shown="真" "回复背景色标志" {
          selector: "回复背景色标志" -> [_ w608]
          frame False {
          }
          frame True {
            w605 = -2 ("Column")
            n342 = Not(x=w608) -> (.not. x?=w607:bool)
            n343 = local write "回复背景色标志"(w607) -> ()
            n344 = Bundle("Column"=w605, "Column"=w605) -> (w606:cluster{"Column":i32, "Column":i32})  [unwired: 1 in]
            n345 = property on="实时数据" class="MCListbox (严格)"("CellBG"=u32 16448250, "ActiveCell"=w606) -> (error out=w604:errorcluster)  [unwired: 2 in, 1 out]
            n346 = Bundle("Column"=-1, "Column"=-2) -> (w601:cluster{"Column":i32, "Column":i32})  [unwired: 1 in]
            n347 = property on="实时数据" class="MCListbox (严格)"(error in=w604, "CellBG"=u32 13816530, "ActiveCell"=w601) -> ()  [unwired: 1 in, 2 out]
          }
        }
      }
      frame True {
        w610 = -2 ("Column")
        w615 = u8 20 ("B动态范围")
        # "处于编辑模式的列表，背景色渐变"
        n348 = local write "回复背景色标志"(w613) -> ()
        n349 = feedback #1(0.0 ("y")) -> (w623:dbl)
        n350 = Greater Or Equal?(x=w623, y=1.0) -> (x >= y?=w618:bool)
        n351 = feedback #2(0.05 ("y")) -> (w621:dbl)
        n352 = Add(x=w623, y=w621) -> (x+y=w626:dbl)
        n353 = feedback-in #1(w626) -> ()
        n354 = case shown="假" w618 {
          tunnel: [w635 -0.05 ("y")] -> w620
          tunnel: w623 -> [w638 _]
          tunnel: w621 -> [w636 _]
          frame False {
            n355 = Less Or Equal?(x=w638, y=-1.0) -> (x <= y?=w634:bool)
            n356 = case shown="真" w634 {
              tunnel: w636 -> [w639 _]
              tunnel: [w639 0.05 ("y")] -> w635
              frame False {
              }
              frame True {
                # "-1"
                n357 = Wait (ms)(milliseconds to wait=u32 0 ("等待时间（毫秒）")) -> ()  [unwired: 1 out]
              }
            }
          }
          frame True {
            # "1"
            n358 = Wait (ms)(milliseconds to wait=u32 0 ("等待时间（毫秒）")) -> ()  [unwired: 1 out]
          }
        }
        n359 = Multiply(x=3.141592653589793, y=w626) -> (x*y=w628:dbl)
        n360 = Cosine(x=w628) -> (cos(x)=w629:dbl)
        n361 = Multiply(x=w629, y=w615) -> (x*y=w619:dbl)
        n362 = Add(x=w619, y=w615) -> (x+y=w617:dbl)
        n363 = Absolute Value(x=w617) -> (abs(x)=w630:dbl)
        n364 = case shown="假" "T:G,F:B" {
          tunnel: w630 -> [w645 w649]
          tunnel: [w646 w648] -> w632
          tunnel: [w644 w647] -> w631
          frame False {
            w646 = u8 255 ("G")
            # "B"
            n365 = Subtract(x=w646, y=w645) -> (x-y=w644:dbl)
          }
          frame True {
            w647 = u8 255 ("G")
            # "G"
            n366 = Subtract(x=w647, y=w649) -> (x-y=w648:dbl)
          }
        }
        n367 = feedback-in #2(w620) -> ()
        n368 = call <vilib>:"RGB to Color.vi"("B"=w632, "G"=w631, "R"=u8 125 ("R常量")) -> ("Color"=w614:u32)
        n369 = Bundle("Column"=w610, "Column"=w610) -> (w611:cluster{"Column":i32, "Column":i32})  [unwired: 1 in]
        n370 = local write "等待时间（毫秒）"(u32 0 ("等待时间（毫秒）")) -> ()
        n371 = property on="实时数据" class="MCListbox (严格)"("CellBG"=w614, "ActiveCell"=w611) -> ()  [unwired: 2 in, 2 out]
      }
    }
    n372 = local read "退出"() -> (w596:bool)
  }
